vi "N7(problems).vi"() -> ()   [LabVIEW 2020]
panel:
  in  "Hige OX":dbl
  in  "Long":i32
  in  "Hige":dbl
  in  "Line 2":dbl[](array[numeric])
  out "Waveform Graph":dbl[][](graph)
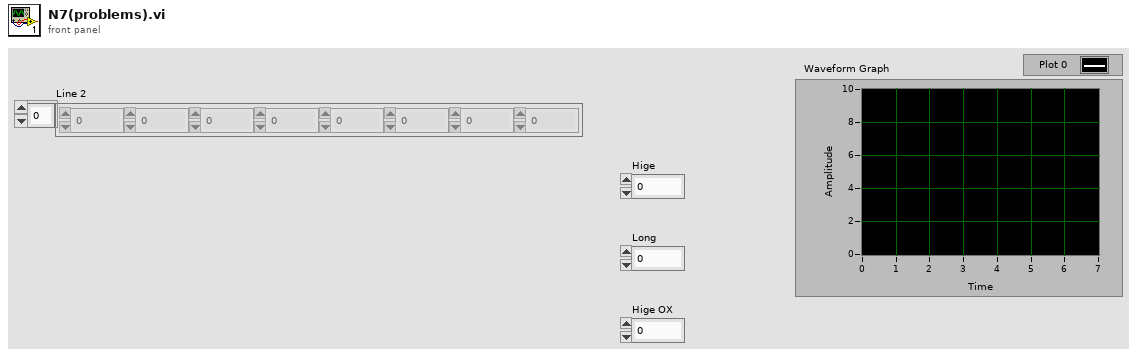
[diagram p1: front panel]
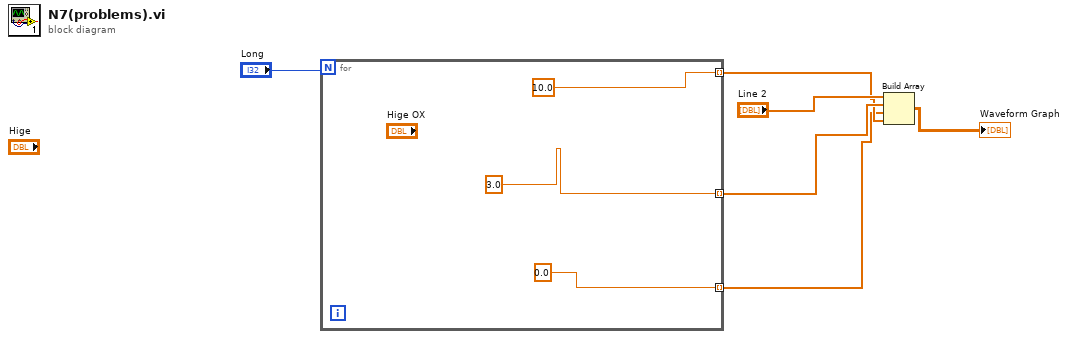
[diagram p0: block diagram]
diagram:
  n1 = for {
    N: "Long" -> [_]
    tunnel: [3.0 ("Hige OX")] -> w5 mode=indexing
    tunnel: [10.0] -> w2 mode=indexing
    tunnel: [0.0] -> w1 mode=indexing
  }
  n2 = Build Array("Line 2", w5, w1, w2) -> (→"Waveform Graph":dbl[][])
